vi "Promass.vi"() -> ()   [LabVIEW 2023]
uses:
  <vilib>/Instr/_visa.llb/VISA Configure Serial Port (Instr).vi
  <vilib>/Utility/file.llb/Write Delimited Spreadsheet (DBL).vi
  <vilib>/ethernetip/ethernetip.lvlib
panel:
  in  "VISA Calibratore":refnum<visa-resource-name>
  in  "Seriale":string
  in  "file path (dialog if empty)":path
  in  "Save Button":bool
  out "Array - Numeric":dbl[][](array[numeric])
  in  "Record Button":bool
  out "Densità [Kg/l]":sgl
  out "Frequenza[Hz]":dbl
  out "Volume [l/min]":sgl
  out "Mass  [Kg/h]":sgl
  out "Temperatura[°C]":sgl
  in  "stop":bool
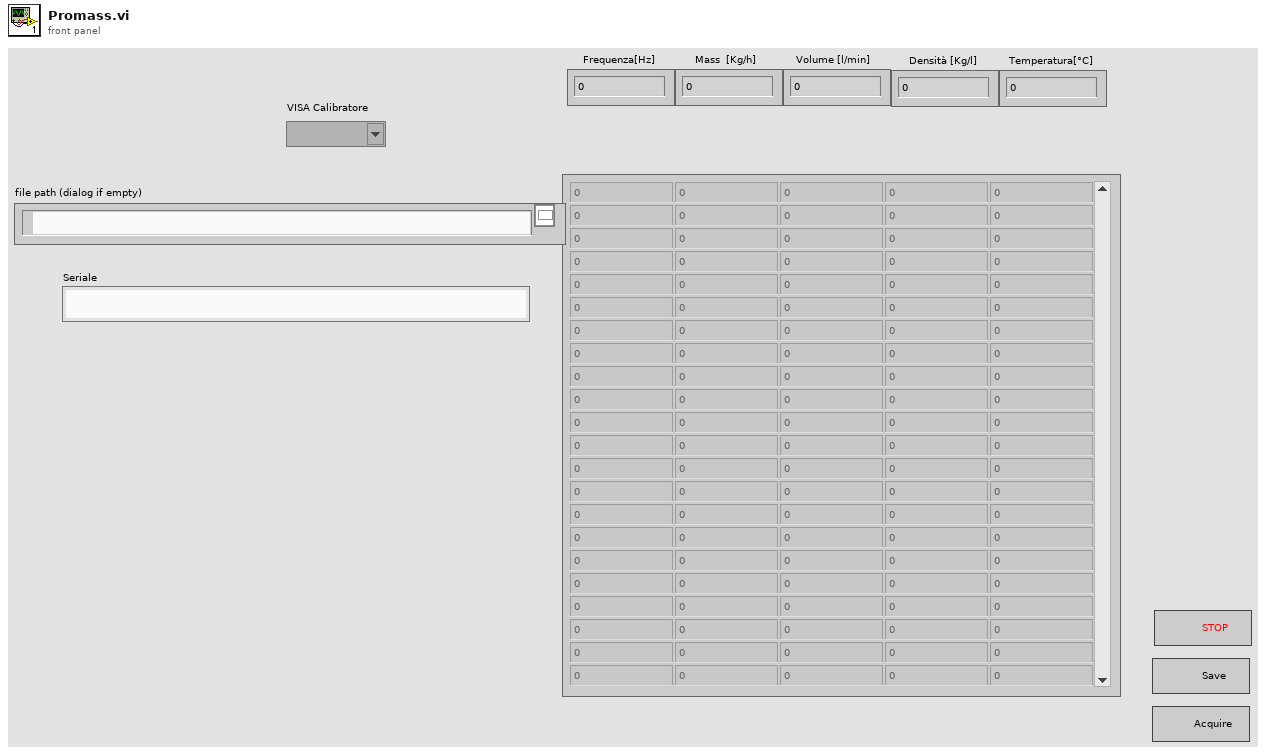
[diagram p1: front panel]
types:
  T1 = enum16{"open", "replace", "create", "open or create", "replace or create", "replace or create with confirmation"}
  T2 = cluster{"Temperatura[°C]":sgl, "Mass  [Kg/h]":sgl, "Volume [l/min]":sgl, "Densità [Kg/l]":sgl, "Pressione [Bar]":dbl, "Frequenza[Hz]":dbl}[]
  T3 = typedef "ethernetip.lvlib/ethernetip.ctl" = refnum<k21>
  T4 = cluster{"Temperatura[°C]":sgl, "Mass  [Kg/h]":sgl, "Volume [l/min]":sgl, "Densità [Kg/l]":sgl, "Pressione [Bar]":dbl, "Frequenza[Hz]":dbl}
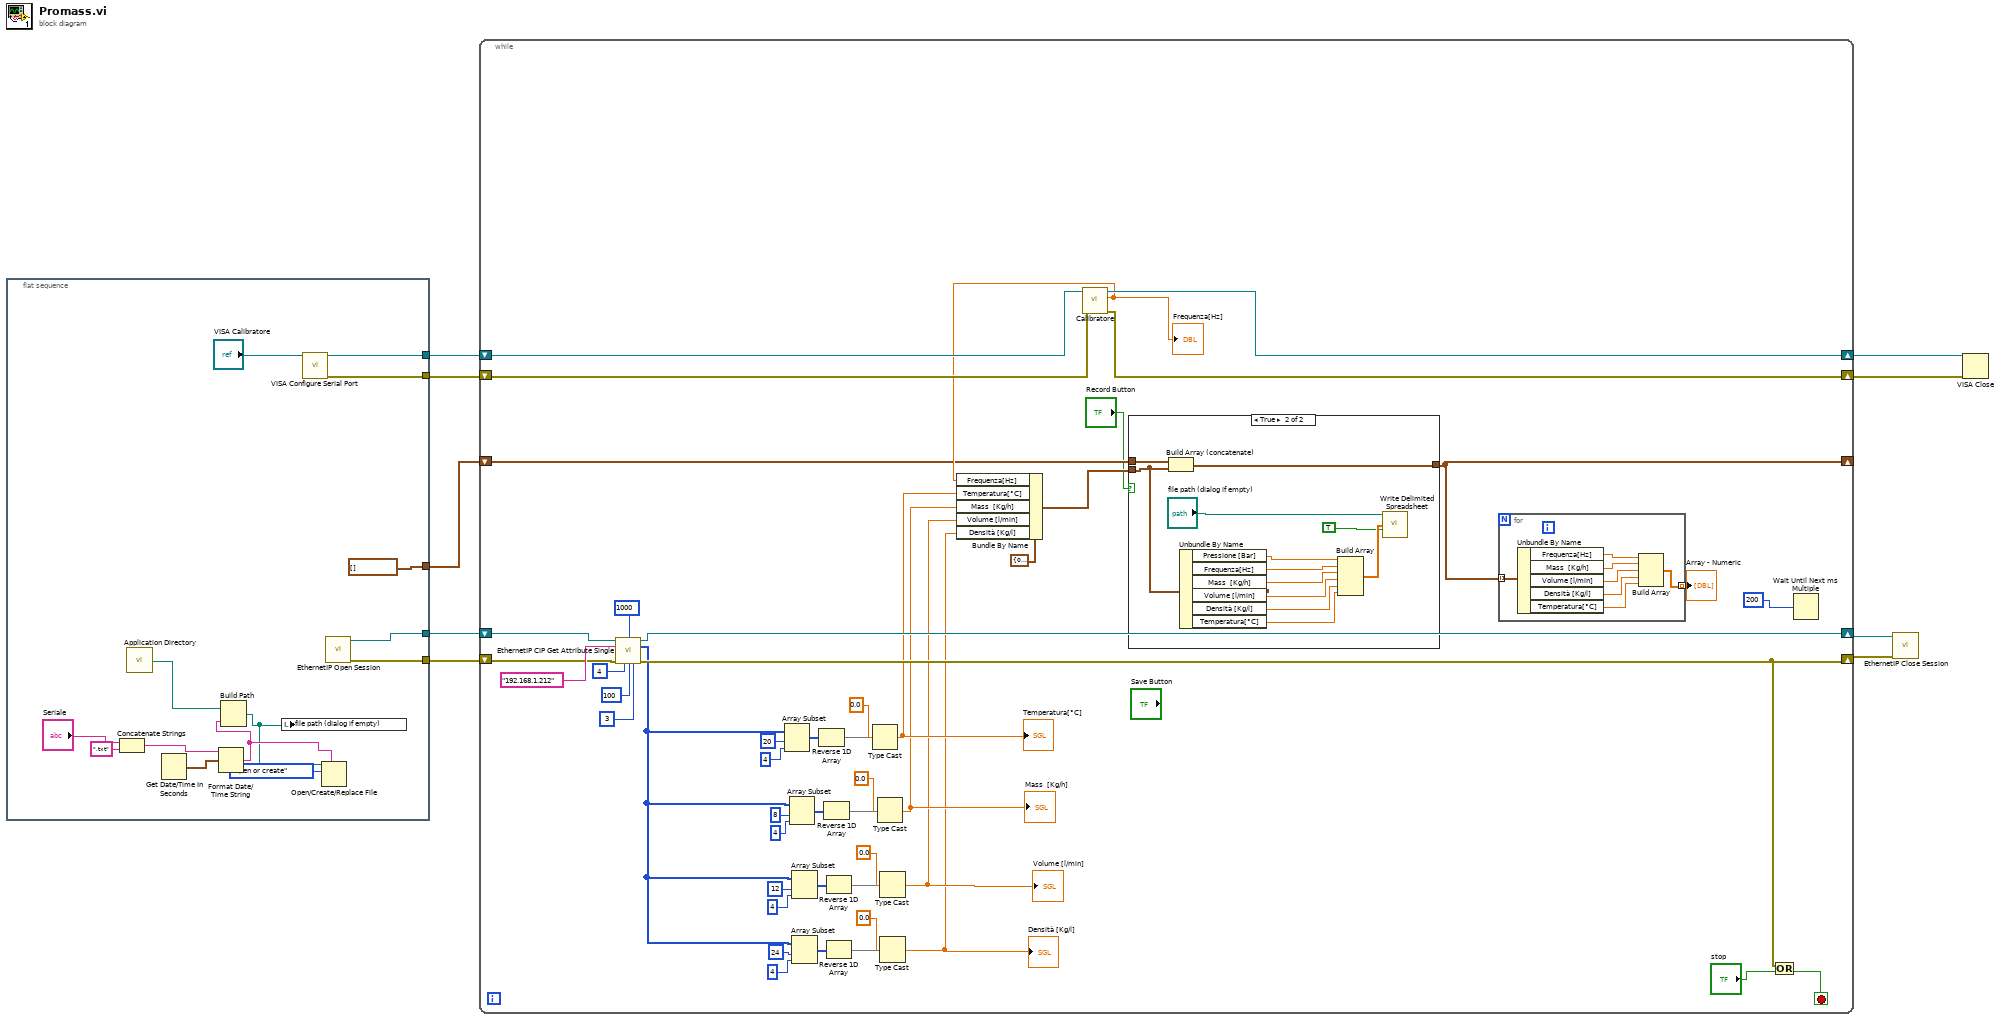
[diagram p0: block diagram]
diagram:
  n1 = flat-sequence {
    tunnel: [w23] -> w7
    tunnel: [w22] -> w6
    tunnel: [w21] -> w5
    tunnel: [w20] -> w3
    tunnel: [T2 []] -> w1
    frame #0 {
      n2 = Concatenate Strings("Seriale", ".txt" ("string")) -> (w15:string)
      n3 = call <vilib>:"Application Directory.vi"() -> ("Application Directory"=w17:path)
      n4 = Get Date/Time In Seconds() -> (seconds since 1Jan1904=w18:timestamp)
      n5 = Format Date/Time String(time format string (%c)=w15, seconds (now)=w18) -> (date/time string=w13:string)  [unwired: 1 in]
      n6 = Build Path(base path=w17, name or relative path=w13) -> (appended path=w12:path)
      n7 = local write "file path (dialog if empty)"(w12) -> ()
      n8 = call-poly "VISA Configure Serial Port"("VISA resource name"="VISA Calibratore") -> ("VISA resource name out"=w21:refnum<visa-resource-name>, "error out"=w20:errorcluster)  [unwired: 13 in]
      n9 = Open/Create/Replace File(file path (use dialog)=w12, prompt=w13, operation (0:open)=T1."open or create") -> ()  [unwired: 3 in, 3 out]
      n10 = call <vilib>:"EthernetIP Open Session.vi"() -> ("error out"=w22:errorcluster, "Session out"=w23:T3)  [unwired: 10 in]
    }
  }
  n11 = while {
    shift-right: [w43] -> w4
    shift-left: w5 -> [w44]
    shift-right: [w64] -> w9
    shift-left: w7 -> [w61]
    shift-right: [w62] -> w8
    shift-left: w6 -> [w60]
    shift-right: [w41] -> w2
    shift-left: w3 -> [w42]
    shift-right: [w25] -> _
    shift-left: w1 -> [w28]
    stop <- w63 stop-if-true
    n12 = call <vilib>:"EthernetIP CIP Get Attribute Single.vi"("Session in"=w61, "Timeout (ms)"=1000, "Network Path"="192.168.1.212", "error in"=w60, "Class"=4, "Instance"=u32 100, "Attribute"=3 ("Class")) -> ("Session out"=w64:T3, "Data"=w38:u8[], "error out"=w62:errorcluster)  [unwired: 6 in]
    n13 = Array Subset(array=w38, index=20, length=4) -> (w55:u8[])
    n14 = Array Subset(array=w38, index=8, length=4) -> (w54:u8[])
    n15 = Array Subset(array=w38, index=12, length=4) -> (w45:u8[])
    n16 = Array Subset(array=w38, index=24, length=4) -> (w35:u8[])
    n17 = Reverse 1D Array(array=w55) -> (reversed array=w56:u8[])
    n18 = Reverse 1D Array(array=w54) -> (reversed array=w53:u8[])
    n19 = Reverse 1D Array(array=w45) -> (reversed array=w46:u8[])
    n20 = Reverse 1D Array(array=w35) -> (reversed array=w37:u8[])
    n21 = Type Cast(type=sgl 0.0, x=w56) -> (*(type *) &x=w32:sgl)
    "Temperatura[°C]" <- w32
    n22 = Type Cast(type=sgl 0.0, x=w53) -> (*(type *) &x=w31:sgl)
    "Mass  [Kg/h]" <- w31
    n23 = Type Cast(type=sgl 0.0, x=w46) -> (*(type *) &x=w30:sgl)
    "Volume [l/min]" <- w30
    n24 = Type Cast(type=sgl 0.0, x=w37) -> (*(type *) &x=w29:sgl)
    "Densità [Kg/l]" <- w29
    n25 = call "Calibratore.vi"("error in (no error)"=w42, "VISA Refnum in"=w44) -> ("error out"=w41:errorcluster, "value"=w33:dbl, "VISA Refnum out"=w43:refnum<visa-resource-name>)  [unwired: 7 in]
    "Frequenza[Hz]" <- w33
    n26 = Bundle By Name(cluster=T4 {"Temperatura[°C]"=0.0, "Mass  [Kg/h]"=0.0, "Volume [l/min]"=0.0, "Densità [Kg/l]"=0.0, "Pressione [Bar]"=0.0, "Frequenza[Hz]"=0.0}, "Frequenza[Hz]"=w33, "Temperatura[°C]"=w32, "Mass  [Kg/h]"=w31, "Volume [l/min]"=w30, "Densità [Kg/l]"=w29) -> (w27:T4)
    n27 = case shown="True" "Record Button" {
      tunnel: w28 -> [w79 w91]
      tunnel: w27 -> [_ w82]
      tunnel: [w79 w90] -> w25
      frame False {
      }
      frame True {
        n28 = Build Array (concatenate)(w91, w82) -> (w90:T2)
        n29 = Unbundle By Name(w82) -> ("Pressione [Bar]"=w83:dbl, "Frequenza[Hz]"=w84:dbl, "Mass  [Kg/h]"=w85:sgl, "Volume [l/min]"=w86:sgl, "Densità [Kg/l]"=w87:sgl, "Temperatura[°C]"=w88:sgl)
        n30 = Build Array(w83, w84, w85, w86, w87, w88) -> (w81:dbl[])
        n31 = call-poly <vilib>:"Write Delimited Spreadsheet.vi"("file path (dialog if empty)"="file path (dialog if empty)", "1D data"=w81, "append to file? (new file:F)"=TRUE) -> ()  [unwired: 11 in, 2 out]
      }
    }
    n32 = for {
      tunnel: w25 -> [w78] mode=indexing
      tunnel: [w72] -> w24 mode=indexing
      n33 = Unbundle By Name(w78) -> ("Frequenza[Hz]"=w77:dbl, "Mass  [Kg/h]"=w76:sgl, "Volume [l/min]"=w75:sgl, "Densità [Kg/l]"=w74:sgl, "Temperatura[°C]"=w73:sgl)
      n34 = Build Array(w77, w76, w75, w74, w73) -> (w72:dbl[])
    }
    "Array - Numeric" <- w24
    n35 = Or(x=w62, y="stop") -> (x .or. y?=w63:bool)
    n36 = Wait Until Next ms Multiple(millisecond multiple=u32 200) -> ()  [unwired: 1 out]
  }
  n37 = call <vilib>:"EthernetIP Close Session.vi"("error in"=w8, "Session in"=w9) -> ()  [unwired: 9 in, 1 out]
  n38 = VISA Close(VISA resource name=w4, error in (no error)=w2) -> ()  [unwired: 1 out]
